vi "HardwareAbortGlobal.vi"(7 "Action":T1=enum."Get", 11 "Set Value":bool) -> (3 "Value Out":bool)   [LabVIEW 2012]
uses:
  HardwareAbortGlobalAction.ctl
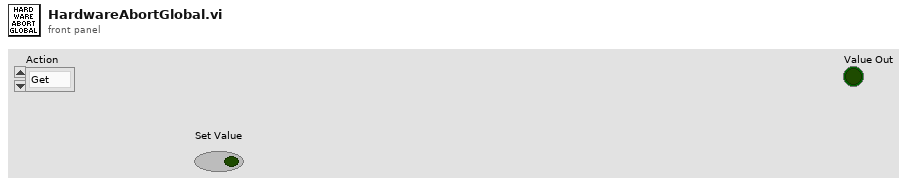
[diagram p1: front panel]
types:
  T1 = typedef "HardwareAbortGlobalAction.ctl" = enum16{"Set", "Get"}
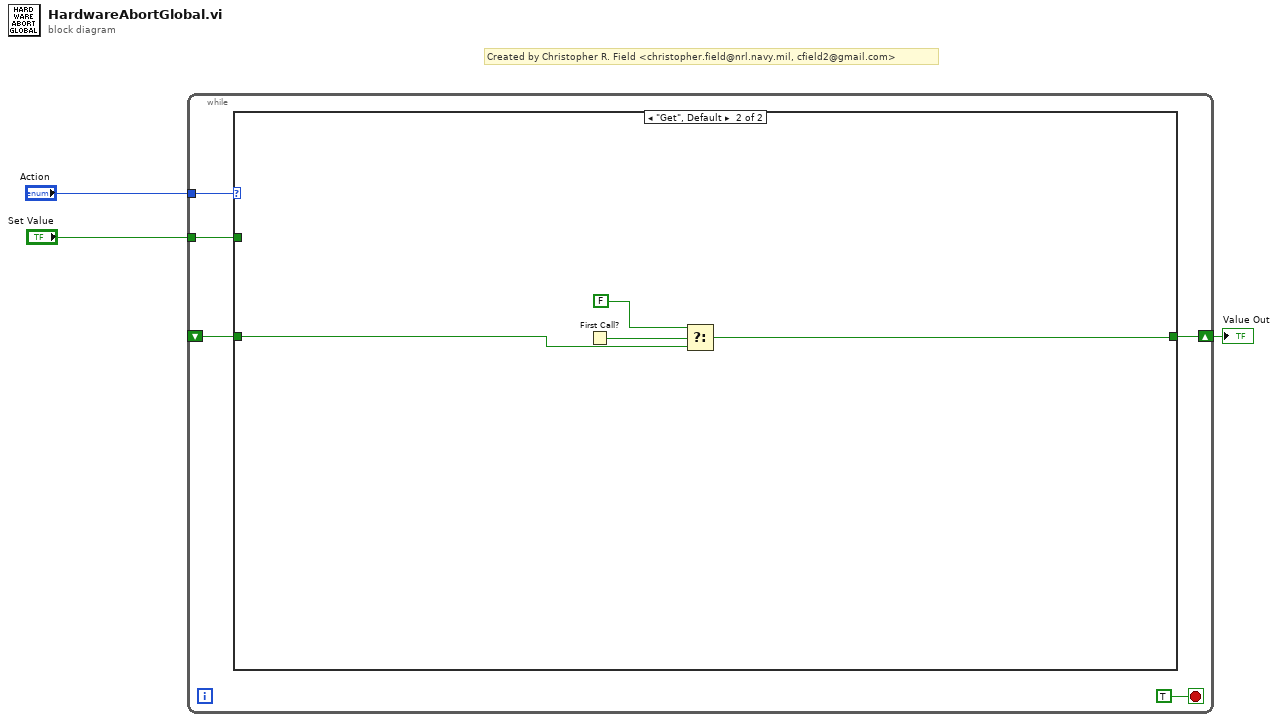
[diagram p0: block diagram]
diagram:
  # "Created by Christopher R. Field <christopher.field@nrl.navy.mil, cfield2@gmail.com>"
  n1 = while {
    tunnel: "Action" -> [w8]
    shift-right: [w6] -> w1
    shift-left: _ -> [w5]
    tunnel: "Set Value" -> [w4]
    stop <- TRUE stop-if-true
    n2 = case shown="\"Get\", Default" w8 {
      tunnel: [w9 w11] -> w6
      tunnel: w5 -> [_ w10]
      tunnel: w4 -> [w9 _]
      frame "Set" {
      }
      frame "Get", Default {
        n3 = First Call?() -> (First Call?: T/F=w13:bool)
        n4 = Select(t=FALSE, s=w13, f=w10) -> (s? t:f=w11:bool)
      }
    }
  }
  "Value Out" <- w1
